vi "SwitchBoard_ChannelMapping.vi"(1 "Sensor type":T1(ring)) -> (0 "subarray":i32[](array[numeric]))   [LabVIEW 2016]
panel:
  # "Some map files are in C:\\Users\\Administrator\\cernbox\\HGCAL test results\\Software\\python\\config"
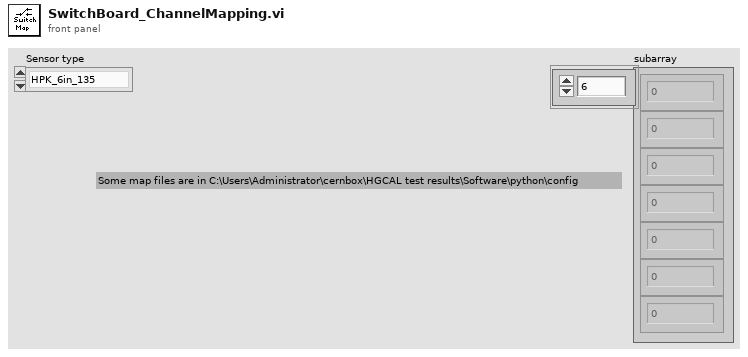
[diagram p1: front panel]
types:
  T1 = enum16{"HPK_6in_135", "HPK_8in_256", "INF_8in_256", "Diode", "HPK_6in_256", "Test capacitances"}
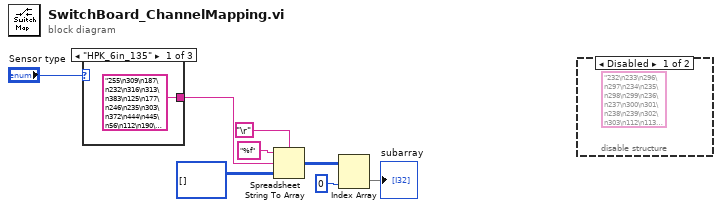
[diagram p0: block diagram]
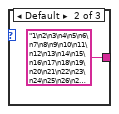
[diagram p3: hidden frame]
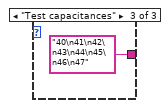
[diagram p4: hidden frame]
diagram:
  n1 = case shown="\"HPK_6in_135\"" "Sensor type" {
    tunnel: ["255\n309\n187\n232\n316\n313\n383\n125\n177\n246\n235\n303\n372\n444\n445\n56\n112\n190\n189\n234\n318\n301\n375\n432\n508\n511\n58\n124\n127\n176\n254\n233\n311\n374\n442\n447\n498\n509\n60\n114\n188\n191\n236\n314\n317\n373\n434\n506\n503\n61\n126\n119\n178\n252\n245\n297\n382\n440\n439\n500\n507\n62\n113\n186\n185\n247\n298\n319\n371\n436\n504\n505\n59\n118\n123\n179\n250\n253\n306\n380\n377\n437\n502\n501\n57\n115\n182\n248\n249\n237\n299\n369\n438\n441\n499\n120\n116\n121\n181\n240\n251\n312\n378\n379\n435\n510\n497\n122\n117\n180\n238\n241\n308\n315\n368\n446\n443\n496\n184\n183\n242\n239\n302\n376\n381\n433\n244\n243\n304\n307\n370\n300\n305\n310\n296\n40\n41\n42\n43\n44\n45\n46\n47\n63\n48\n49\n50\n51\n52\n53\n54\n55" "1\n2\n3\n4\n5\n6\n7\n8\n9\n10\n11\n12\n13\n14\n15\n16\n17\n18\n19\n20\n21\n22\n23\n24\n25\n26\n27\n28\n29\n30\n31\n32\n33\n34\n35\n36\n37\n38\n39\n40\n41\n42\n43\n44\n45\n46\n47\n48\n49\n50\n51\n52\n53\n54\n55\n56\n57\n58\n59\n60\n61\n62\n63\n64\n65\n66\n67\n68\n69\n70\n71\n72\n73\n74\n75\n76\n77\n78\n79\n80\n81\n82\n83\n84\n85\n86\n87\n88\n89\n90\n91\n92\n93\n94\n95\n96\n97\n98\n99\n100\n101\n102\n103\n104\n105\n106\n107\n108\n109\n110\n111\n112\n113\n114\n115\n116\n117\n118\n119\n120\n121\n122\n123\n124\n125\n126\n127\n128\n129\n130\n131\n132\n133\n134\n135\n136\n137\n138\n139\n140\n141\n142\n143\n144\n145\n146\n147\n148\n149\n150\n151\n152\n153\n154\n155\n156\n157\n158\n159\n160\n161\n162\n163\n164\n165\n166\n167\n168\n169\n170\n171\n172\n173\n174\n175\n176\n177\n..." "40\n41\n42\n43\n44\n45\n46\n47"] -> w8
    frame "HPK_6in_135" {
    }
    frame Default {
    }
    frame "Test capacitances" {
    }
  }
  n2 = Spreadsheet String To Array(delimiter (Tab)="\r", format string="%f", spreadsheet string=w8, array type (2D Dbl)=i32[][] []) -> (array=w4:i32[][])
  n3 = Index Array(array=w4, index (col)=0 ("index (row)")) -> (element=→"subarray":i32[])  [unwired: 1 in]
  n4 = disable-structure shown="Disabled" {
    frame Disabled {
      (unwired) "232\n233\n296\n297\n234\n235\n298\n299\n236\n237\n300\n301\n238\n239\n302\n303\n112\n113\n176\n177\n240\n241\n305\n304\n368\n369\n432\n433\n496\n497\n114\n115\n178\n179\n242\n243\n307\n306\n370\n371\n434\n435\n498\n499\n116\n117\n180\n181\n244\n245\n309\n308\n372\n373\n436\n437\n500\n501\n118\n119\n182\n183\n246\n247\n311\n310\n374\n375\n438\n439\n502\n503\n56\n57\n121\n184\n248\n249\n313\n126\n185\n312\n376\n377\n440\n441\n504\n505\n58\n59\n123\n186\n250\n251\n315\n124\n187\n314\n378\n379\n442\n443\n506\n507\n60\n61\n125\n188\n252\n253\n317\n122\n189\n316\n380\n381\n444\n445\n508\n509\n62\n127\n190\n254\n255\n319\n120\n191\n318\n382\n383\n446\n447\n510\n511\n40\n41\n43\n42\n44\n45\n46\n47"
    }
    frame Enabled {
    }
  }
